vi "Build Preview.vi"(7 "Ambient":dbl, 8 "error in (no error)":errorcluster, 9 "Start Temp":dbl, 10 "Start Time":dbl, 11 "Recipe Step in":refnum<class "Recipe Step.lvclass">) -> (0 "error out":errorcluster, 1 "End Temp":dbl, 2 "End Time":dbl, 3 "Recipe Step out":refnum<class "Recipe Step.lvclass">, 4 "Step Plot Data":cluster{"Time":dbl[], "Value":dbl[]})   [LabVIEW 2018, in "Temp Recipe.lvlib" / "Recipe Step.lvclass"]
uses:
  Recipe Step.lvclass
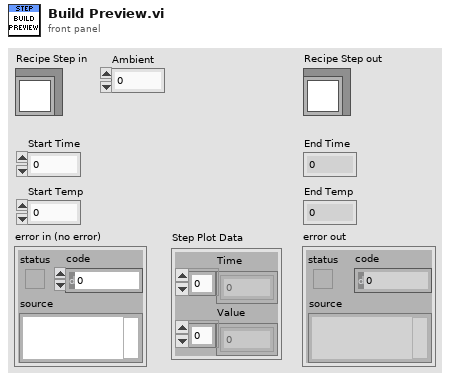
[diagram p1: front panel]
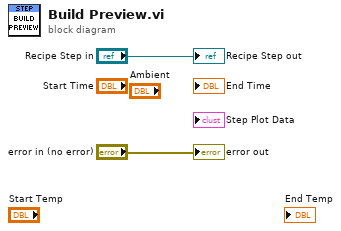
[diagram p0: block diagram]
diagram:
  "error out" <- "error in (no error)"
  "Recipe Step out" <- "Recipe Step in"
